vi "Launch New AUT Instance.vi"(8 "error in (no error)":errorcluster, 11 "Test Harness in":refnum<class "Business Logic Tester.lvclass">) -> (0 "error out":errorcluster, 3 "Test Harness out":refnum<class "Business Logic Tester.lvclass">)   [LabVIEW 2020, in "Business Logic Tester.lvlib" / "Business Logic Tester.lvclass"]
uses:
  Business Logic Tester.lvclass
  C:/Program Files (x86)/National Instruments/LabVIEW 2020/vi.lib/ActorFramework/Actor/Actor.lvclass
  Business Logic/Business Logic/Business Logic.lvclass
  Business Logic Tester.lvclass/Business Logic Tester.ctl
  <vilib>/ActorFramework/Message Enqueuer/Init from Existing Queue.vi
  <vilib>/ActorFramework/Message Enqueuer/Message Enqueuer.lvclass
  <vilib>/ActorFramework/Actor/Actor.lvclass
  <vilib>/SAS/Actor Tester/Enqueuer Manager/SAS_AFTester_Enqueuer Manager.lvclass
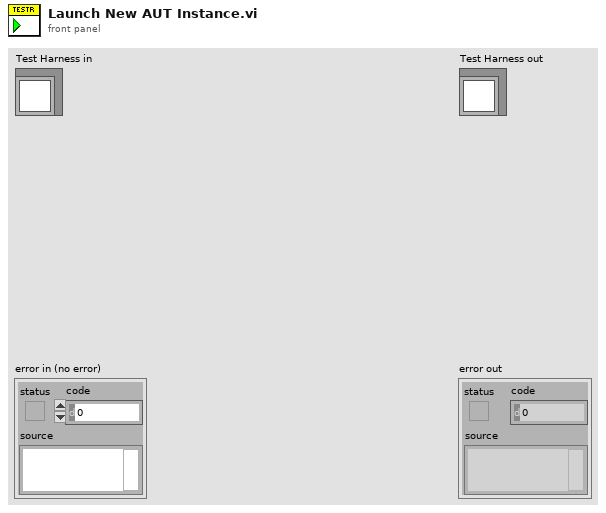
[diagram p1: front panel]
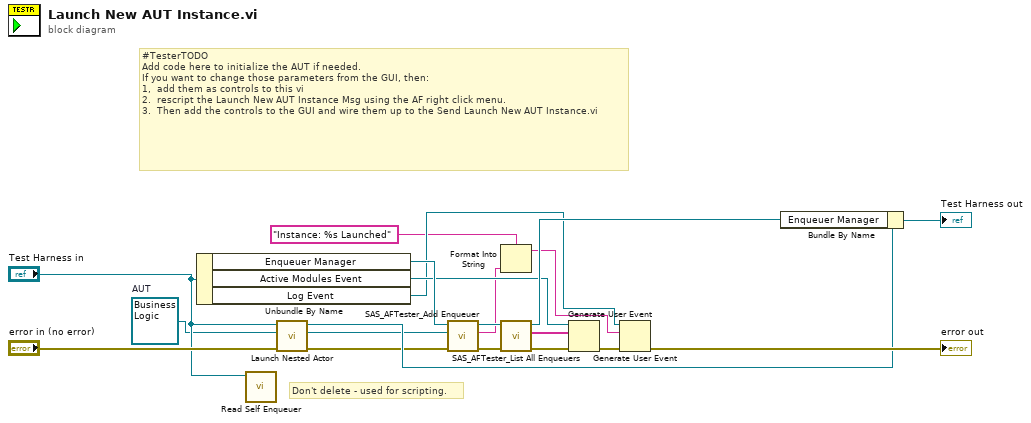
[diagram p0: block diagram]
diagram:
  w16 = refnum<class "Business Logic.lvclass"> refnum  # AUT
  # "Don't delete - used for scripting."
  # "#TesterTODO\nAdd code here to initialize the AUT if needed.\nIf you want to change those parameters from the GUI, then:\n1,  add them as controls to this vi \n2.  rescript the Launch New AUT Instance Msg using the AF right click menu.  \n3.  Then add the controls to the GUI and wire them up to the Send Launch New AUT Instance.vi"
  n1 = Unbundle By Name("Test Harness in") -> ("Enqueuer Manager"=w14:refnum<class "SAS_AFTester_Enqueuer Manager.lvclass">, "Active Modules Event"=w8:refnum<user-event>, "Log Event"=w4:refnum<user-event>)
  n2 = call <vilib>:"Read Self Enqueuer.vi"("Actor"="Test Harness in") -> ()  [unwired: 10 in, 1 out]
  n3 = call <vilib>:"Launch Nested Actor.vi"("error in (no error)"="error in (no error)", "Nested Actor"=w16, "Caller Actor in"="Test Harness in") -> ("error out"=w13:errorcluster, "Nested Actor's Enqueuer"=w12:refnum<class "Message Enqueuer.lvclass">, "Caller Actor out"=w15:refnum<class "Business Logic Tester.lvclass">)  [unwired: 6 in]
  n4 = call <vilib>:"SAS_AFTester_Add Enqueuer.vi"("error in (no error)"=w13, "Message Enqueuer"=w12, "Enqueuer Manager in"=w14) -> ("error out"=w10:errorcluster, "Enqueuer ID"=w1:string, "Enqueuer Manager out"=w11:refnum<class "SAS_AFTester_Enqueuer Manager.lvclass">)  [unwired: 6 in]
  n5 = Format Into String(format string="Instance: %s Launched" ("event data"), w1) -> (resulting string=w3:string)  [unwired: 2 in, 1 out]
  n6 = call <vilib>:"SAS_AFTester_List All Enqueuers.vi"("error in (no error)"=w10, "Enqueuer Manager in"=w11) -> ("error out"=w6:errorcluster, "All Enqueuers"=w7:string[], "Enqueuer Manager out"=w9:refnum<class "SAS_AFTester_Enqueuer Manager.lvclass">)  [unwired: 7 in]
  n7 = Generate User Event(user event=w8, event data cluster=w7, error in=w6) -> (error out=w5:errorcluster)  [unwired: 1 in, 1 out]
  n8 = Generate User Event(user event=w4, event data cluster=w3, error in=w5) -> (error out=→"error out":errorcluster)  [unwired: 1 in, 1 out]
  n9 = Bundle By Name(cluster=w15, "Enqueuer Manager"=w9) -> (→"Test Harness out":refnum<class "Business Logic Tester.lvclass">)
